vi "Fs_to_FilterDelay.vi"(11 "Fs":u32) -> (3 "Total Filter Delay (samples)":u32)   [LabVIEW 2020, in "DAQmx.AI.lvclass"]
uses:
  DAQmx.AI.lvclass
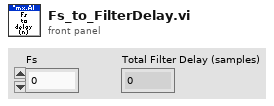
[diagram p1: front panel]
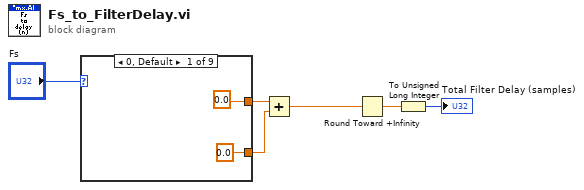
[diagram p0: block diagram]
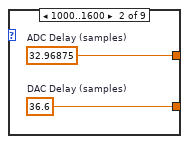
[diagram p2: hidden frame]
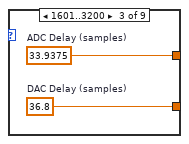
[diagram p3: hidden frame]
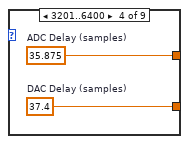
[diagram p4: hidden frame]
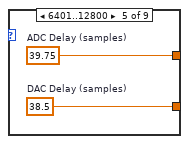
[diagram p5: hidden frame]
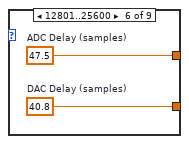
[diagram p6: hidden frame]
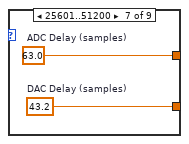
[diagram p7: hidden frame]
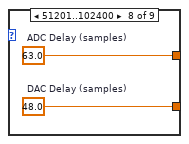
[diagram p8: hidden frame]
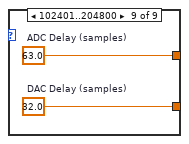
[diagram p9: hidden frame]
diagram:
  n1 = case shown="0, Default" "Fs" {
    tunnel: [0.0 ("ADC Delay (samples)") w10 w12 w14 w16 w18 w20 w22 w24] -> w5
    tunnel: [0.0 ("ADC Delay (samples)") w9 w11 w13 w15 w17 w19 w21 w23] -> w4
    frame 0, Default {
    }
    frame 1000..1600 {
      w9 = 36.6  # DAC Delay (samples)
      w10 = 32.96875  # ADC Delay (samples)
    }
    frame 1601..3200 {
      w11 = 36.8  # DAC Delay (samples)
      w12 = 33.9375  # ADC Delay (samples)
    }
    frame 3201..6400 {
      w13 = 37.4  # DAC Delay (samples)
      w14 = 35.875  # ADC Delay (samples)
    }
    frame 6401..12800 {
      w15 = 38.5  # DAC Delay (samples)
      w16 = 39.75  # ADC Delay (samples)
    }
    frame 12801..25600 {
      w17 = 40.8  # DAC Delay (samples)
      w18 = 47.5  # ADC Delay (samples)
    }
    frame 25601..51200 {
      w20 = 63.0  # ADC Delay (samples)
      w19 = 43.2  # DAC Delay (samples)
    }
    frame 51201..102400 {
      w22 = 63.0  # ADC Delay (samples)
      w21 = 48.0  # DAC Delay (samples)
    }
    frame 102401..204800 {
      w24 = 63.0  # ADC Delay (samples)
      w23 = 32.0  # DAC Delay (samples)
    }
  }
  n2 = Add(x=w5, y=w4) -> (x+y=w3:dbl)
  n3 = Round Toward +Infinity(x=w3) -> (ceil(x): smallest int >= x=w2:dbl)
  n4 = To Unsigned Long Integer(number=w2) -> (unsigned 32bit integer=→"Total Filter Delay (samples)":u32)
